vi "Complex Test.vi"() -> ()   [LabVIEW 2020, in "infolib.lvlib"]
doc: "Make a complex test of the library using premade tests/test.info."
uses:
  infolib.lvlib
  Get key polymorph parts/GetString.vi
  Add key polymorph parts/String.vi
  Get matrix polymorph parts/Get 2D String.vi
  Add matrix polymorph parts/2D String.vi
  Get key polymorph parts/GetTime Stamp.vi
  Add key polymorph parts/Time Stamp.vi
  Get matrix polymorph parts/Get 2D Time Stamp.vi
  Add matrix polymorph parts/2D Time Stamp.vi
  Get key polymorph parts/GetEXT.vi
  Add key polymorph parts/EXT.vi
  Get key polymorph parts/GetCXT.vi
  Add key polymorph parts/CXT.vi
  Get matrix polymorph parts/Get 2D EXT.vi
  Add matrix polymorph parts/2D EXT.vi
  Get matrix polymorph parts/Get 2D CXT.vi
  Add matrix polymorph parts/2D CXT.vi
  <vilib>/Utility/error.llb/Error Cluster From Error Code.vi
  <vilib>/ErrorRing/Error Ring.xnode
panel:
  in  "error limit for time":dbl=1e-06 format="%#_13g"
  in  "error limit for double":ext=1e-12
  in  "Test definitions and correct values":T1(array[cluster])=[{"k"="Test key, no value", "v"=[[""]], "t"="string", "s"=[]}, {"k"="Test key", "v"=[["A"]], "t"="string", "s"=[]}, {"k"="Test key, similar", "v"=[["B"]], "t"="string", "s"=[]}, {"k"="Test key, no spaces", "v"=[["C"]], "t"="string", "s"=[]}, {"k"="Test key, both spaces", "v"=[["D"]], "t"="string", "s"=[]}, {"k"="Test key, space left", "v"=[["E"]], "t"="string", "s"=[]}, {"k"="Test key, space right", "v"=[["F"]], "t"="string", "s"=[]}, {"k"="Test integer, 16 digits", "v"=[["1234567890123456"]], "t"="number", "s"=[]}, {"k"="Test floating point, 16 digits after decimal dot", "v"=[["0.1234567890123456"]], "t"="number", "s"=[]}, {"k"="Test floating point, 15 digits before decimal dot", "v"=[["123456789012345.6"]], "t"="number", "s"=[]}, {"k"="Test complex number", "v"=[["2.34+5.67i"]], "t"="compl. number", "s"=[]}, {"k"="Test imaginary number", "v"=[["8.90i"]], "t"="compl. number", "s"=[]}, {"k"="Test string, simple", "v"=[["test string"]], "t"="string", "s"=[]}, {"k"="Test string, nonletter characters", "v"=[["!@#$%^&*()-=[]{};'\"\\'\\\"\\:|,./<>?"]], "t"="string", "s"=[]}, {"k"="Test string, nonletter characters in key !@#$%^&*()-=[]{};'\"\\'\\\"\\:|,./<>?", "v"=[["in key"]], "t"="string", "s"=[]}, {"k"="Test string, UTF8 characters", "v"=[["\\u0159\\u0153\\u0414\\u03bc\\u03a9\\u211c\\u2111"]], "t"="string", "s"=[]}, {"k"="Test string, UTF8 characters in key \\u0159\\u0153\\u0414\\u03bc\\u03a9\\u211c\\u2111", "v"=[["in key"]], "t"="string", "s"=[]}, {"k"="Test time, no time zone", "v"=[["1014376332.123456"]], "t"="time", "s"=[]}, {"k"="Test time, with time zone, UTC", "v"=[["1014379932.123456"]], "t"="time", "s"=[]}, {"k"="Test time, with time zone, +10 minutes", "v"=[["1014379932.123456"]], "t"="time", "s"=[]}, {"k"="Test time, with time zone, +1 hour", "v"=[["1014379932.123456"]], "t"="time", "s"=[]}, {"k"="Test time, with time zone, -1 hour", "v"=[["1014379932.123456"]], "t"="time", "s"=[]}, {"k"="Test time, with time zone, +1:10", "v"=[["1014379932.123456"]], "t"="time", "s"=[]}, {"k"="Test time, with time zone, -1:10", "v"=[["1014379932.123456"]], "t"="time", "s"=[]}, {"k"="Test matrix, empty", "v"=[[""]], "t"="matrix number", "s"=[]}, {"k"="Test matrix, single value", "v"=[["1"]], "t"="matrix number", "s"=[]}, {"k"="Test matrix, single value, nonletter characters in key !@#$%^&*()-=[]{};'\"\\'\\\"\\:|,./<>?", "v"=[["2"]], "t"="matrix number", "s"=[]}, {"k"="Test matrix, single value, UTF8 characters in key  \\u0159\\u0153\\u0414\\u03bc\\u03a9\\u211c\\u2111", "v"=[["3"]], "t"="matrix number", "s"=[]}, {"k"="Test matrix, row numbers", "v"=[["4", "5", "6"]], "t"="matrix number", "s"=[]}, {"k"="Test matrix, column numbers", "v"=[["7"], ["8"], ["9"]], "t"="matrix number", "s"=[]}, {"k"="Test matrix", "v"=[["1.1", "2.1", "3.1"], ["4e4", "-5e5", "6e-6"], ["7.7e7", "8.123456789e1", "NaN"]], "t"="matrix number", "s"=[]}, {"k"="Test matrix complex", "v"=[["1.234", "2.345i", "3.456+4.567i"]], "t"="matrix compl. number", "s"=[]}, {"k"="Test matrix, mixed numbers and text for reading as numbers", "v"=[["1", "NaN", "2", "NaN"], ["3", "NaN", "4", "NaN"]], "t"="matrix number", "s"=[]}, {"k"="Test matrix, mixed numbers and text for reading as strings", "v"=[["11", "One", "12", "Two"], ["13", "Three", "14", "Four"]], "t"="matrix string", "s"=[]}, {"k"="Test matrix, mixed numbers and text with special characters read as numbers", "v"=[["1", "NaN", "2", "NaN"], ["3", "NaN", "4", "NaN"]], "t"="matrix number", "s"=[]}, {"k"="Test matrix, mixed numbers and text with special characters read as strings", "v"=[["11", "One;One", "12", "Two\"Two"], ["13", "Three;Three", "14", "Four\n                Four"]], "t"="matrix string", "s"=[]}, {"k"="Test matrix, time values", "v"=[["1014379932.123456", "1014383532.123456"], ["1014387132.123456", "1014390732.123456"]], "t"="matrix time", "s"=[]}, {"k"="Test matrix, lousy format and spaces", "v"=[["77", "8.8", "NaN"], ["NaN", "999", "10"], ["11", "12", "13"]], "t"="matrix number", "s"=[]}, {"k"="Key for section test", "v"=[["1"]], "t"="number", "s"=[""]}, {"k"="Key for section test", "v"=[["2"]], "t"="number", "s"=["Test section"]}, {"k"="Key for section test", "v"=[["3"]], "t"="number", "s"=["Test section", "Test subsection"]}, {"k"="Key for section test", "v"=[["4"]], "t"="number", "s"=["Test section", "Test subsection", "Test subsubsection"]}, {"k"="Key for section test", "v"=[["5"]], "t"="number", "s"=["Test section", "Test subsection", "Test subsubsection", "Test subsubsubsection"]}, {"k"="Key for section test", "v"=[["6"]], "t"="number", "s"=["Test section 2"]}, {"k"="Key for section test", "v"=[["7"]], "t"="number", "s"=["Test section 2", "Test section 2"]}, {"k"="Key for section test", "v"=[["8"]], "t"="number", "s"=["Test section 2", "Test section 2", "Test section 2"]}, {"k"="Key for section test", "v"=[["9"]], "t"="number", "s"=["Test section 2", "Test section 2", "Test section 2", "Test section 2"]}, {"k"="Key for section test", "v"=[["10"]], "t"="number", "s"=["Test section, nonletter characters in key !@#$%^&*()-=[]{};'\"\\'\\\"\\:|,./<>?"]}, {"k"="Key for section test", "v"=[["11"]], "t"="number", "s"=["Test section, UTF8 characters in key \\u0159\\u0153\\u0414\\u03bc\\u03a9\\u211c\\u2111"]}, {"k"="Key for section test", "v"=[["!@#$%^&*()-=[]{};'\"\\'\\\"\\:|,./<>?"]], "t"="section", "s"=["Test section, special characters inside"]}]
  in  "Do also tmp.info?":bool=TRUE
  in  "start:":i32
  in  "end:":i32=100
  out "tmp.info: all correct?":bool
  out "tmp.info: all keys found?":bool
  out "Results of testing":T2(array[cluster])
  out "test.info: all keys found?":bool
  out "test.info: all correct?":bool
  # "k: key, v: value of correct value, t: test type, s: section(s)"
  # "For details see \"tests/info_test.m\" and \"tests/test.info\"."
  # "Do not change values in the array without changing test.info and other testing scripts (infolib_test.m)!"
  # "First run from test.info"
  # "test index, test key, key found?, test correct?"
  # "Second run from generated tmp.info"
  # "For debugging: do tests only from index"
  # "to index"
  # "(inclusive), do tmp.info"
  # "<- To make full test, set values to 0 and 100 and check tmp.info."
  # "List of bad tests, with very small impact:\n15, 16, 27, 47, 48: LV cannot handle UTF8 characters\n43: fails if tests 47 and 48 are present in tmp.info, otherwise is ok.\n30: rounding error on 17th significant place\n34,:LV cannot handle proper csv: cell \"X;X\" is considered as two cells because LV do not know apostroph enclosing\n36: rounding error on 7th decimal place of time stamp"
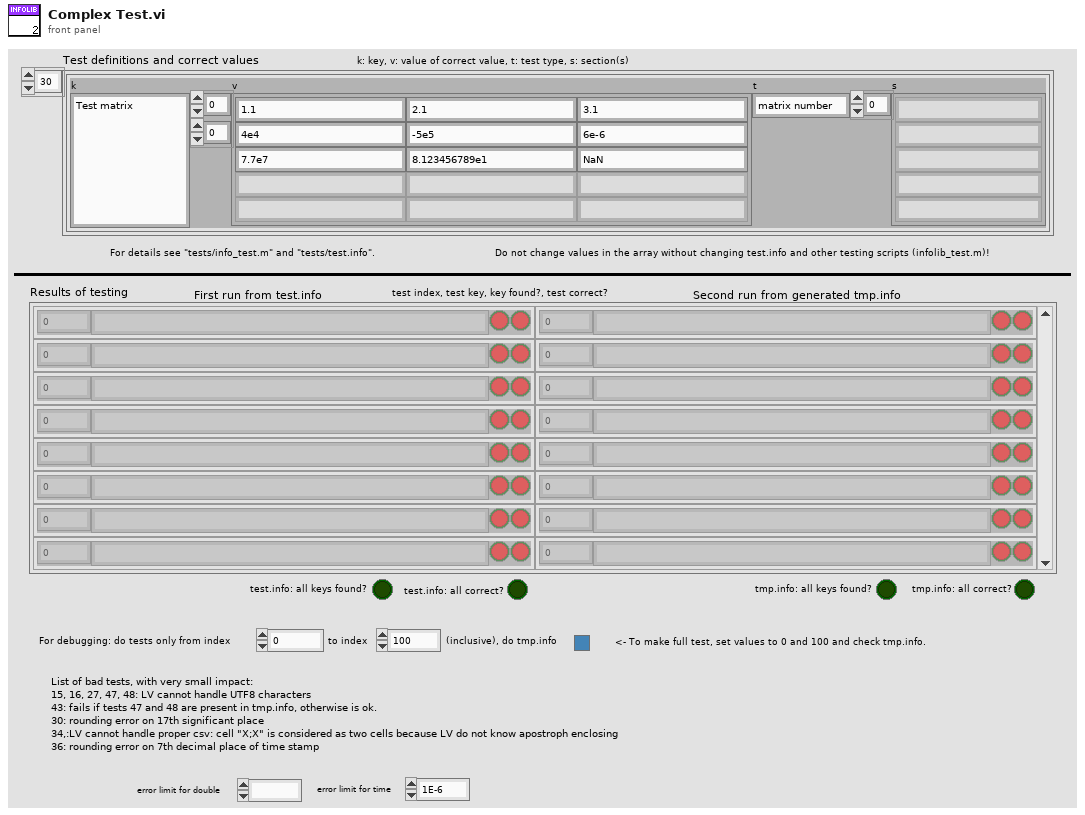
[diagram p1: front panel]
types:
  T1 = cluster{"k":string, "v":string[][], "t":string, "s":string[]}[]
  T2 = cluster{"index":i32, "key":string, "key found?":bool, "correct?":bool}[][]
  T3 = cluster{"index":i32, "key":string, "key found?":bool, "correct?":bool}
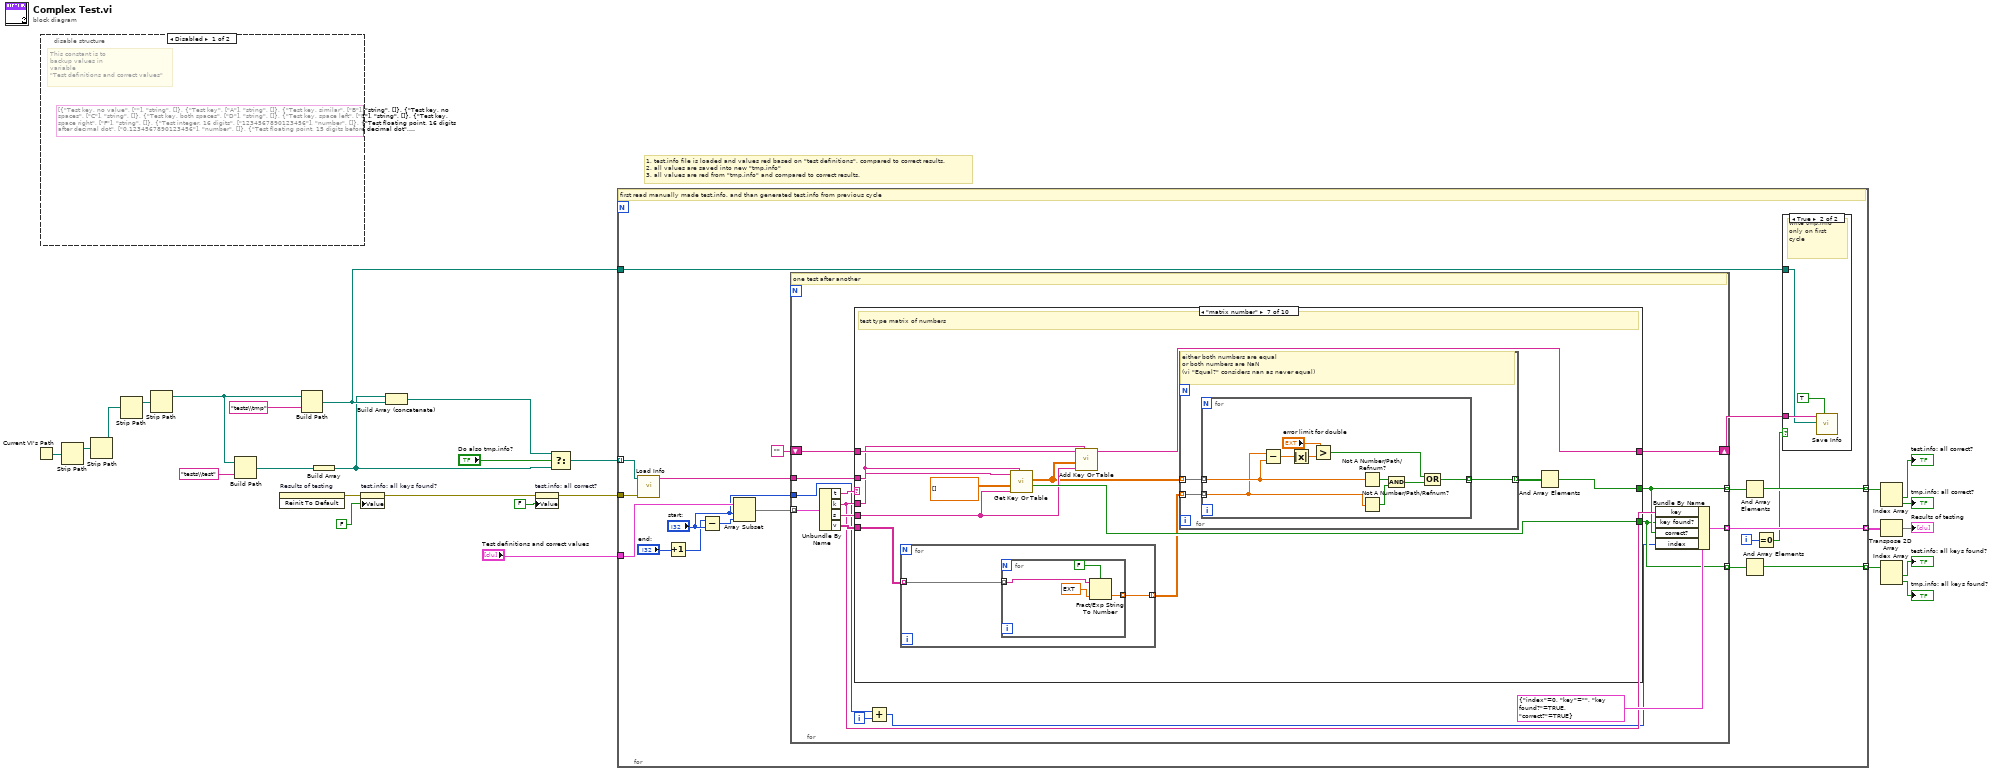
[diagram p0: block diagram]
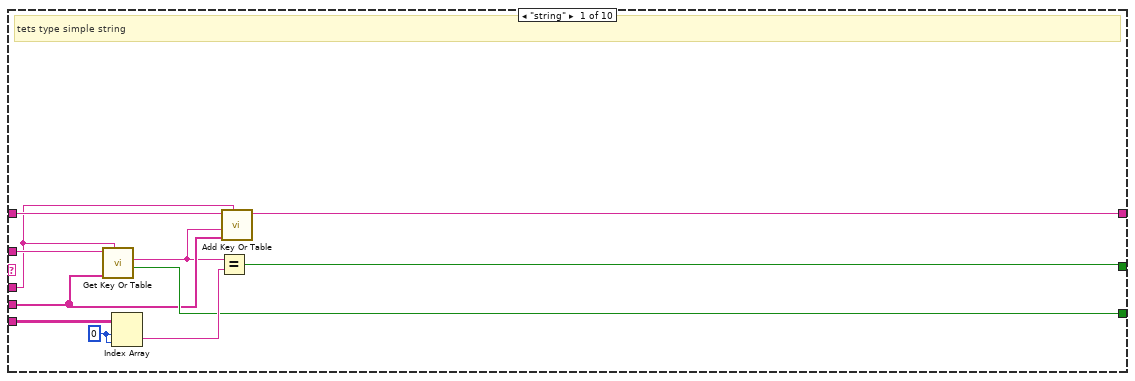
[diagram p3: hidden frame]
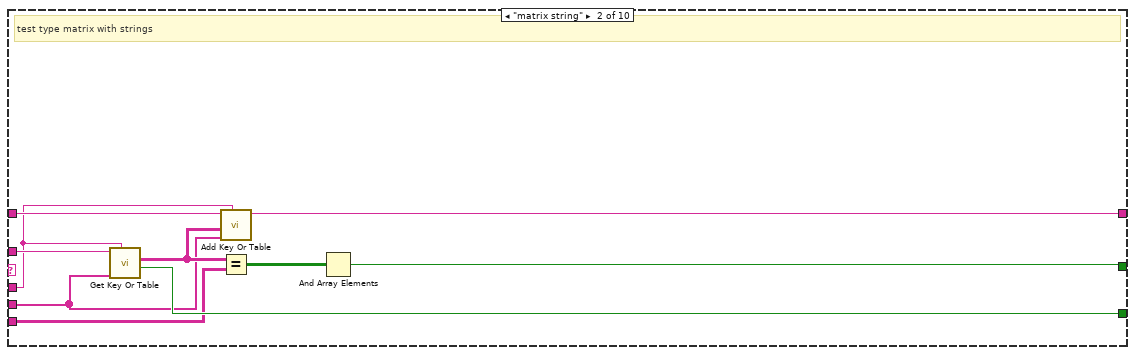
[diagram p4: hidden frame]
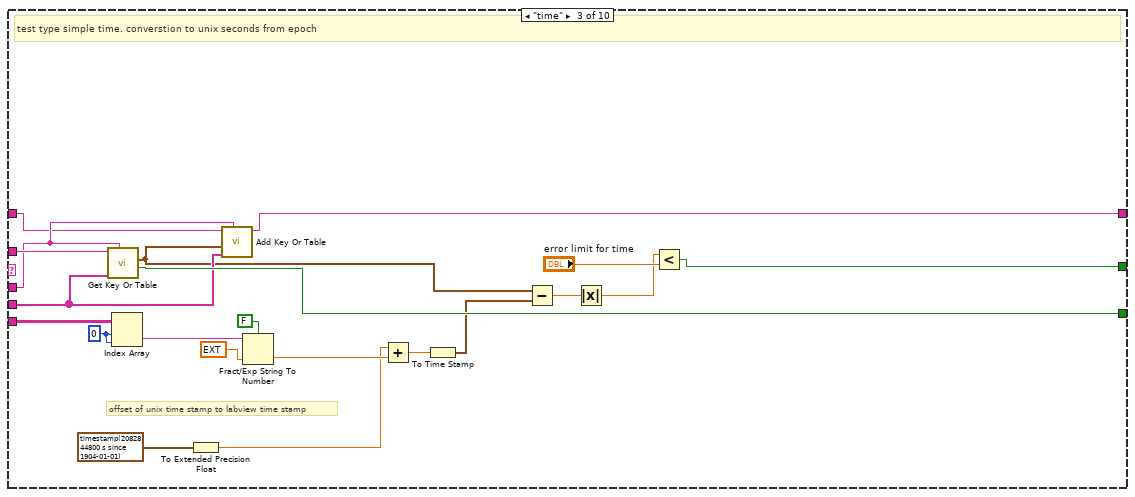
[diagram p5: hidden frame]
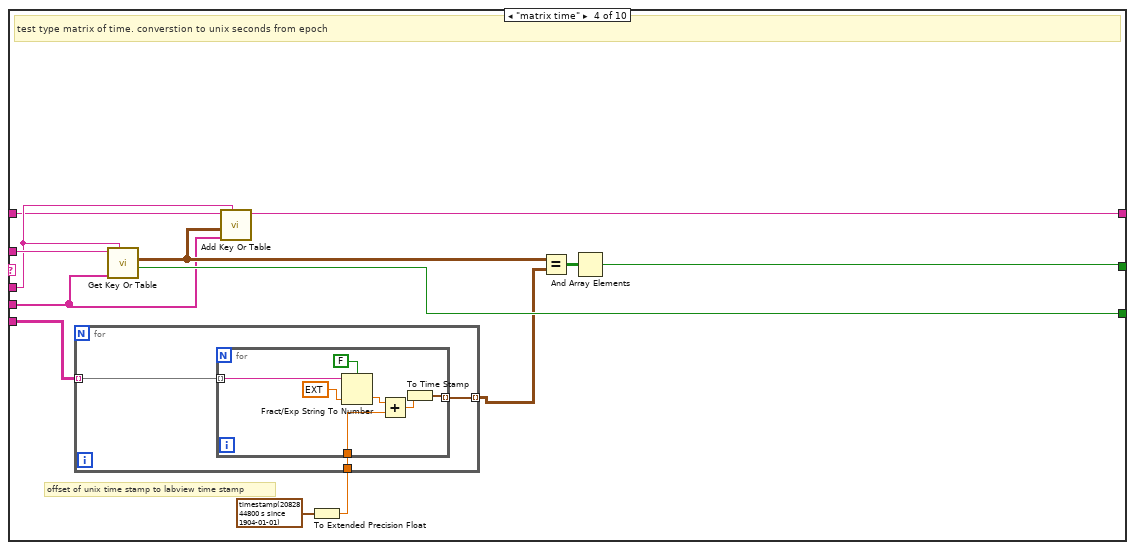
[diagram p6: hidden frame]
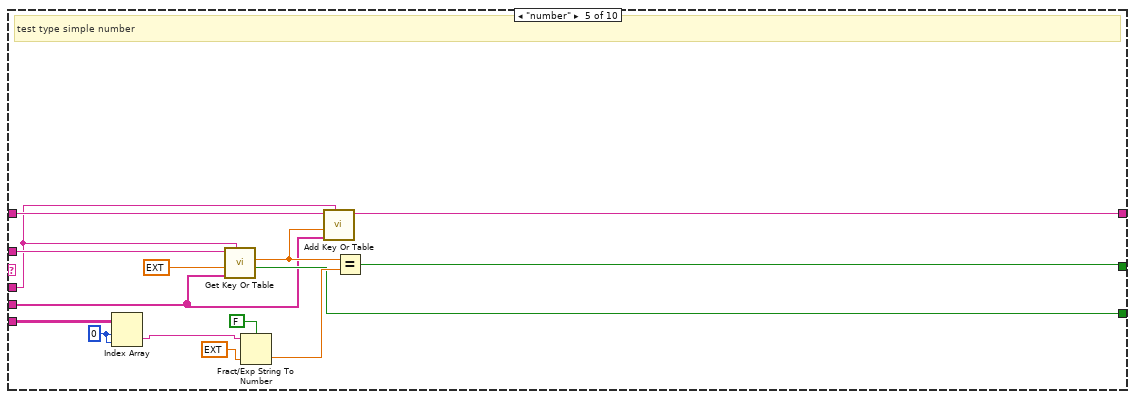
[diagram p7: hidden frame]
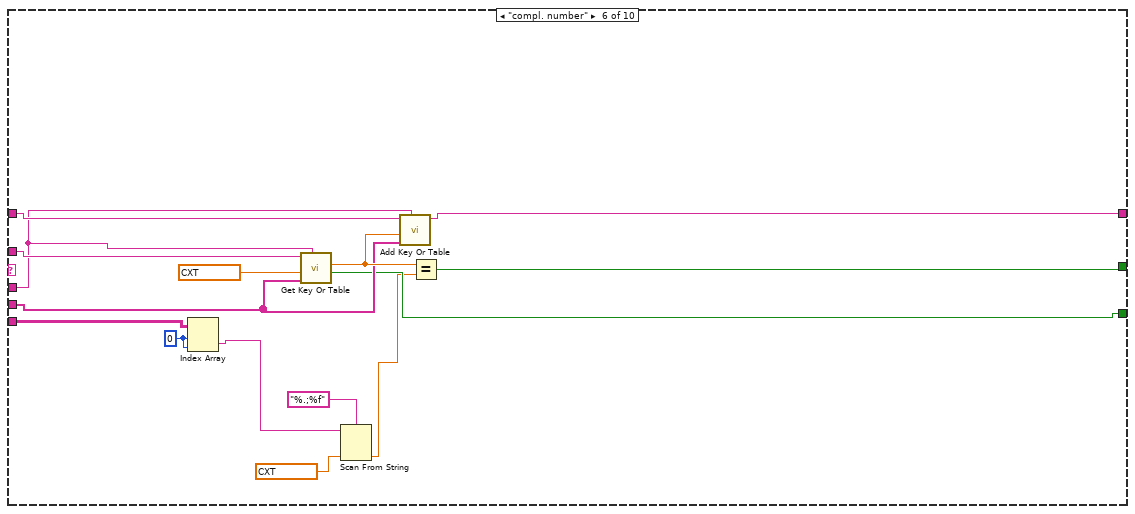
[diagram p8: hidden frame]
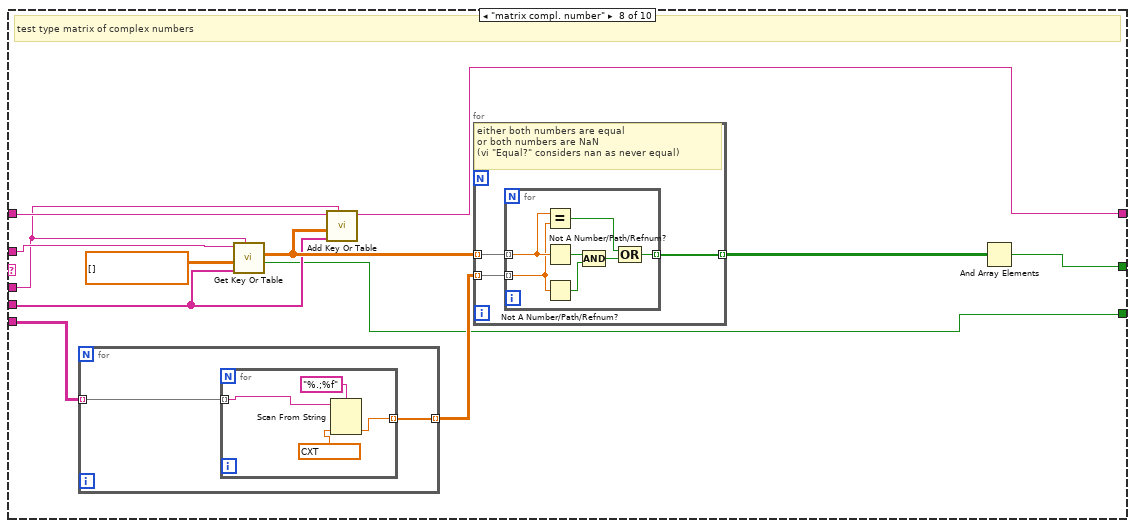
[diagram p9: hidden frame]
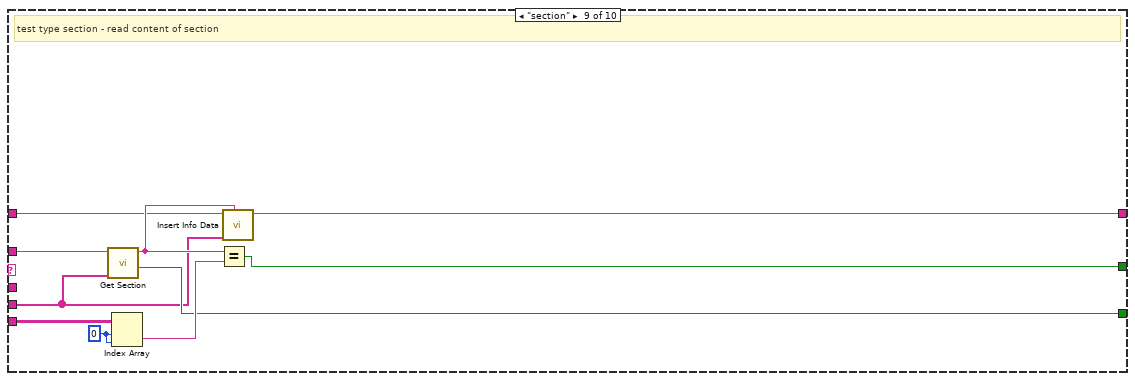
[diagram p10: hidden frame]
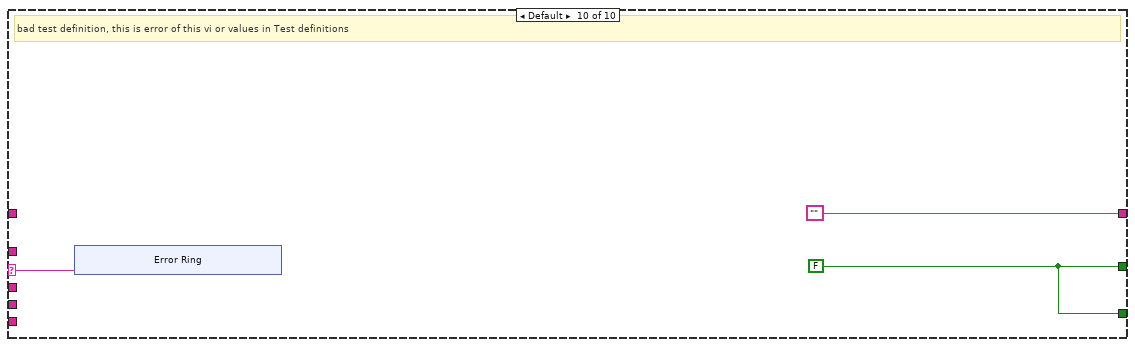
[diagram p11: hidden frame]
diagram:
  # "1, test.info file is loaded and values red based on \"test definitions\", compared to correct results.\n2, all values are saved into new \"tmp.info\"\n3, all values are red from \"tmp.info\" and compared to correct results."
  n1 = Current VI's Path() -> (path=w15:path)
  n2 = disable-structure shown="Disabled" {
    frame Disabled {
      (unwired) T1 [{"k"="Test key, no value", "v"=[[""]], "t"="string", "s"=[]}, {"k"="Test key", "v"=[["A"]], "t"="string", "s"=[]}, {"k"="Test key, similar", "v"=[["B"]], "t"="string", "s"=[]}, {"k"="Test key, no spaces", "v"=[["C"]], "t"="string", "s"=[]}, {"k"="Test key, both spaces", "v"=[["D"]], "t"="string", "s"=[]}, {"k"="Test key, space left", "v"=[["E"]], "t"="string", "s"=[]}, {"k"="Test key, space right", "v"=[["F"]], "t"="string", "s"=[]}, {"k"="Test integer, 16 digits", "v"=[["1234567890123456"]], "t"="number", "s"=[]}, {"k"="Test floating point, 16 digits after decimal dot", "v"=[["0.1234567890123456"]], "t"="number", "s"=[]}, {"k"="Test floating point, 15 digits before decimal dot", "v"=[["123456789012345.6"]], "t"="number", "s"=[]}, {"k"="Test complex number", "v"=[["2.34+5.67i"]], "t"="compl. number", "s"=[]}, {"k"="Test imaginary number", "v"=[["8.90i"]], "t"="compl. number", "s"=[]}, {"k"="Test string, simple", "v"=[["test string"]], "t"="string", "s"=[]}, {"k"="Test string, nonletter characters", "v"=[["!@#$%^&*()-=[]{};'\"\\'\\\"\\:|,./<>?"]], "t"="string", "s"=[]}, {"k"="Test string, nonletter characters in key !@#$%^&*()-=[]{};'\"\\'\\\"\\:|,./<>?", "v"=[["in key"]], "t"="string", "s"=[]}, {"k"="Test string, UTF8 characters", "v"=[["\\u0159\\u0153\\u0414\\u03bc\\u03a9\\u211c\\u2111"]], "t"="string", "s"=[]}, {"k"="Test string, UTF8 characters in key \\u0159\\u0153\\u0414\\u03bc\\u03a9\\u211c\\u2111", "v"=[["in key"]], "t"="string", "s"=[]}, {"k"="Test time, no time zone", "v"=[["1014376332.123456"]], "t"="time", "s"=[]}, {"k"="Test time, with time zone, UTC", "v"=[["1014379932.123456"]], "t"="time", "s"=[]}, {"k"="Test time, with time zone, +10 minutes", "v"=[["1014379932.123456"]], "t"="time", "s"=[]}, {"k"="Test time, with time zone, +1 hour", "v"=[["1014379932.123456"]], "t"="time", "s"=[]}, {"k"="Test time, with time zone, -1 hour", "v"=[["1014379932.123456"]], "t"="time", "s"=[]}, {"k"="Test time, with time zone, +1:10", "v"=[["1014379932.123456"]], "t"="time", "s"=[]}, {"k"="Test time, with time zone, -1:10", "v"=[["1014379932.123456"]], "t"="time", "s"=[]}, {"k"="Test matrix, empty", "v"=[[""]], "t"="matrix number", "s"=[]}, {"k"="Test matrix, single value", "v"=[["1"]], "t"="matrix number", "s"=[]}, {"k"="Test matrix, single value, nonletter characters in key !@#$%^&*()-=[]{};'\"\\'\\\"\\:|,./<>?", "v"=[["2"]], "t"="matrix number", "s"=[]}, {"k"="Test matrix, single value, UTF8 characters in key  \\u0159\\u0153\\u0414\\u03bc\\u03a9\\u211c\\u2111", "v"=[["3"]], "t"="matrix number", "s"=[]}, {"k"="Test matrix, row numbers", "v"=[["4", "5", "6"]], "t"="matrix number", "s"=[]}, {"k"="Test matrix, column numbers", "v"=[["7"], ["8"], ["9"]], "t"="matrix number", "s"=[]}, {"k"="Test matrix", "v"=[["1.1", "2.1", "3.1"], ["4e4", "-5e5", "6e-6"], ["7.7e7", "8.123456789e1", "NaN"]], "t"="matrix number", "s"=[]}, {"k"="Test matrix complex", "v"=[["1.234", "2.345i", "3.456+4.567i"]], "t"="matrix compl. number", "s"=[]}, {"k"="Test matrix, mixed numbers and text for reading as numbers", "v"=[["1", "NaN", "2", "NaN"], ["3", "NaN", "4", "NaN"]], "t"="matrix number", "s"=[]}, {"k"="Test matrix, mixed numbers and text for reading as strings", "v"=[["11", "One", "12", "Two"], ["13", "Three", "14", "Four"]], "t"="matrix string", "s"=[]}, {"k"="Test matrix, mixed numbers and text with special characters read as numbers", "v"=[["1", "NaN", "2", "NaN"], ["3", "NaN", "4", "NaN"]], "t"="matrix number", "s"=[]}, {"k"="Test matrix, mixed numbers and text with special characters read as strings", "v"=[["11", "One;One", "12", "Two\"Two"], ["13", "Three;Three", "14", "Four\n                Four"]], "t"="matrix string", "s"=[]}, {"k"="Test matrix, time values", "v"=[["1014379932.123456", "1014379932.123456+1*3600"], ["1014379932.123456+2*3600", "1014379932.123456+3*3600"]], "t"="matrix time", "s"=[]}, {"k"="Key for section test", "v"=[["1"]], "t"="number", "s"=[""]}, {"k"="Key for section test", "v"=[["2"]], "t"="number", "s"=["Test section"]}, {"k"="Key for section test", "v"=[["3"]], "t"="number", "s"=["Test section", "Test subsection"]}, {"k"="Key for section test", "v"=[["4"]], "t"="number", "s"=["Test section", "Test subsection", "Test subsubsection"]}, {"k"="Key for section test", "v"=[["5"]], "t"="number", "s"=["Test section", "Test subsection", "Test subsubsection", "Test subsubsubsection"]}, {"k"="Key for section test", "v"=[["6"]], "t"="number", "s"=["Test section 2"]}, {"k"="Key for section test", "v"=[["7"]], "t"="number", "s"=["Test section 2", "Test section 2"]}, {"k"="Key for section test", "v"=[["8"]], "t"="number", "s"=["Test section 2", "Test section 2", "Test section 2"]}, {"k"="Key for section test", "v"=[["9"]], "t"="number", "s"=["Test section 2", "Test section 2", "Test section 2", "Test section 2"]}, {"k"="Key for section test", "v"=[["10"]], "t"="number", "s"=["Test section, nonletter characters in key !@#$%^&*()-=[]{};'\"\\'\\\"\\:|,./<>?"]}, {"k"="Key for section test", "v"=[["11"]], "t"="number", "s"=["Test section, UTF8 characters in key \\u0159\\u0153\\u0414\\u03bc\\u03a9\\u211c\\u2111"]}, {"k"="Key for section test", "v"=[["!@#$%^&*()-=[]{};'\"\\'\\\"\\:|,./<>?"]], "t"="section", "s"=["Test section, special characters inside"]}] ("Test definitions and correct values")
      # "This constant is to\nbackup values in\nvariable\n\"Test definitions and correct values\""
    }
    frame Enabled {
    }
  }
  n3 = Strip Path(path=w15) -> (stripped path=w14:path)  [unwired: 1 out]
  n4 = Strip Path(path=w14) -> (stripped path=w13:path)  [unwired: 1 out]
  n5 = Strip Path(path=w13) -> (stripped path=w12:path)  [unwired: 1 out]
  n6 = Strip Path(path=w12) -> (stripped path=w11:path)  [unwired: 1 out]
  n7 = Build Path(base path=w11, name or relative path="tests\\test") -> (appended path=w3:path)
  n8 = invoke on="Results of testing" class="Arr (strict)" method="Reinit To Default"() -> (error out=w8:errorcluster)  [unwired: 3 in, 2 out]
  n9 = Build Path(base path=w11, name or relative path="tests\\tmp") -> (appended path=w7:path)
  n10 = Build Array(w3) -> (w2:path[])
  n11 = property on="test.info: all keys found?" class="Bool (strict)"(error in=w8, "Value"=FALSE ("All keys found?")) -> (error out=w27:errorcluster)  [unwired: 1 in, 1 out]
  n12 = Build Array (concatenate)(w2, w7) -> (w4:path[])
  n13 = property on="test.info: all correct?" class="Bool (strict)"(error in=w27, "Value"=FALSE ("All correct?")) -> (error out=w26:errorcluster)  [unwired: 1 in, 1 out]
  n14 = Select(t=w4, s="Do also tmp.info?", f=w2) -> (s? t:f=w6:path[])
  n15 = for {
    tunnel: "Test definitions and correct values" -> [w33]
    tunnel: w6 -> [w46] mode=indexing
    tunnel: w26 -> [w44]
    tunnel: [w43] -> w10 mode=indexing
    tunnel: [w41] -> w17 mode=indexing
    tunnel: [w39] -> w21 mode=indexing
    tunnel: w7 -> [w34]
    i -> [w37]
    # "first read manually made test.info, and than generated test.info from previous cycle"
    n16 = call "Load Info.vi"("error in"=w44, "filename"=w46) -> ("info data"=w45:string)  [unwired: 8 in, 1 out]
    n17 = Increment(x="end:") -> (x+1=w28:i32)
    n18 = Subtract(x=w28, y="start:") -> (x-y=w30:i32)
    n19 = Array Subset(array=w33, index="start:", length=w30) -> (w32:T1)
    n20 = for {
      tunnel: w32 -> [w64] mode=indexing
      tunnel: w45 -> [w63]
      tunnel: [w57] -> w43 mode=indexing
      tunnel: [w56] -> w42 mode=indexing
      tunnel: [w55] -> w40 mode=indexing
      shift-right: [w53] -> w35
      shift-left: "" -> [w54]
      tunnel: "start:" -> [w51]
      i -> [w52]
      # "one test after another"
      n21 = Unbundle By Name(w64) -> ("t"=w62:string, "k"=w58:string, "s"=w61:string[], "v"=w60:string[][])
      n22 = case shown="\"matrix number\"" w62 {
        selector: w62 -> [_ _ _ _ _ _ _ _ _ w230]
        tunnel: w58 -> [w67 w79 w97 w112 w135 w155 w164 w196 _ _]
        tunnel: w63 -> [w75 w85 w106 w119 w144 w156 w171 w197 w228 _]
        tunnel: w61 -> [w69 w77 w96 w109 w133 w153 w163 w195 w220 _]
        tunnel: w60 -> [w74 w83 w105 w116 w143 w154 w168 w194 w227 _]
        tunnel: [w72 w81 w88 w114 w142 w152 w167 w191 w224 w231] -> w56
        tunnel: [w71 w84 w104 w118 w138 w150 w170 w193 w223 w231] -> w55
        tunnel: w54 -> [w70 w80 w95 w111 w136 w157 w166 w198 w221 _]
        tunnel: [w66 w76 w94 w110 w132 w151 w165 w192 w219 ""] -> w53
        frame "string" {
          w65 = 0 ("index (row)")
          # "tets type simple string"
          n23 = call-poly "Get Key Or Table.vi"("key description"=w67, "sections"=w69, "info data"=w75) -> ("key found?"=w71:bool, "value"=w68:string)  [unwired: 5 in, 2 out]
          n24 = Index Array(array=w74, index (row)=w65, index (col)=w65) -> (element=w73:string)
          n25 = Equal?(x=w68, y=w73) -> (x = y?=w72:bool)
          n26 = call-poly "Add Key Or Table.vi"("key description"=w67, "sections"=w69, "string"=w68, "info data"=w70) -> ("info data out"=w66:string)  [unwired: 6 in, 1 out]
        }
        frame "matrix string" {
          # "test type matrix with strings"
          n27 = call-poly "Get Key Or Table.vi"("key description"=w79, "sections"=w77, "info data"=w85) -> ("key found?"=w84:bool, "value"=w78:string[][])  [unwired: 5 in, 2 out]
          n28 = call-poly "Add Key Or Table.vi"("key description"=w79, "sections"=w77, "string"=w78, "info data"=w80) -> ("info data out"=w76:string)  [unwired: 6 in, 1 out]
          n29 = Equal?(x=w78, y=w83) -> (x = y?=w82:bool[][])
          n30 = And Array Elements(Boolean array=w82) -> (logical AND=w81:bool)
        }
        frame "time" {
          w93 = 0 ("index (row)")
          # "offset of unix time stamp to labview time stamp"
          # "test type simple time. converstion to unix seconds from epoch"
          n31 = call-poly "Get Key Or Table.vi"("key description"=w97, "sections"=w96, "info data"=w106) -> ("key found?"=w104:bool, "value"=w90:timestamp)  [unwired: 5 in, 2 out]
          n32 = Index Array(array=w105, index (row)=w93, index (col)=w93) -> (element=w102:string)
          n33 = To Extended Precision Float(1:timestamp(2082844800 s since 1904-01-01)) -> (0:w100:ext)
          n34 = call-poly "Add Key Or Table.vi"("key description"=w97, "sections"=w96, "time stamp"=w90, "info data"=w95) -> ("info data out"=w94:string)  [unwired: 6 in, 1 out]
          n35 = Fract/Exp String To Number(use system decimal point (T)=FALSE, string=w102, default (0 dbl)=ext nan ("default (0 DBL)")) -> (number=w101:ext)  [unwired: 1 in, 1 out]
          n36 = Add(x=w100, y=w101) -> (x+y=w98:ext)
          n37 = To Time Stamp(1:w98) -> (0:w91:timestamp)
          n38 = Subtract(x=w90, y=w91) -> (x-y=w87:dbl)
          n39 = Absolute Value(x=w87) -> (abs(x)=w86:dbl)
          n40 = Less?(x=w86, y="error limit for time") -> (x < y?=w88:bool)
        }
        frame "matrix time" {
          # "offset of unix time stamp to labview time stamp"
          # "test type matrix of time. converstion to unix seconds from epoch"
          n41 = call-poly "Get Key Or Table.vi"("key description"=w112, "sections"=w109, "info data"=w119) -> ("key found?"=w118:bool, "value"=w113:timestamp[][])  [unwired: 5 in, 2 out]
          n42 = call-poly "Add Key Or Table.vi"("key description"=w112, "sections"=w109, "time stamp"=w113, "info data"=w111) -> ("info data out"=w110:string)  [unwired: 6 in, 1 out]
          n43 = To Extended Precision Float(1:timestamp(2082844800 s since 1904-01-01)) -> (0:w107:ext)
          n44 = for {
            tunnel: [w122] -> w108 mode=indexing
            tunnel: w116 -> [w121] mode=indexing
            tunnel: w107 -> [w120]
            n45 = for {
              tunnel: [w124] -> w122 mode=indexing
              tunnel: w121 -> [w128] mode=indexing
              tunnel: w120 -> [w123]
              n46 = Fract/Exp String To Number(use system decimal point (T)=FALSE, string=w128, default (0 dbl)=ext nan ("default (0 DBL)")) -> (number=w126:ext)  [unwired: 1 in, 1 out]
              n47 = Add(x=w126, y=w123) -> (x+y=w125:ext)
              n48 = To Time Stamp(1:w125) -> (0:w124:timestamp)
            }
          }
          n49 = Equal?(x=w113, y=w108) -> (x = y?=w115:bool[][])
          n50 = And Array Elements(Boolean array=w115) -> (logical AND=w114:bool)
        }
        frame "number" {
          w131 = 0 ("index (row)")
          # "test type simple number"
          n51 = Index Array(array=w143, index (row)=w131, index (col)=w131) -> (element=w141:string)
          n52 = call-poly "Get Key Or Table.vi"("key description"=w135, "sections"=w133, "numeric"=ext nan, "info data"=w144) -> ("key found?"=w138:bool, "value"=w134:ext)  [unwired: 4 in, 2 out]
          n53 = Fract/Exp String To Number(use system decimal point (T)=FALSE, string=w141, default (0 dbl)=ext nan ("default (0 DBL)")) -> (number=w140:ext)  [unwired: 1 in, 1 out]
          n54 = call-poly "Add Key Or Table.vi"("key description"=w135, "sections"=w133, "numeric"=w134, "info data"=w136) -> ("info data out"=w132:string)  [unwired: 6 in, 1 out]
          n55 = Equal?(x=w134, y=w140) -> (x = y?=w142:bool)
        }
        frame "compl. number" {
          w158 = 0 ("index (row)")
          n56 = Index Array(array=w154, index (row)=w158, index (col)=w158) -> (element=w147:string)
          n57 = call-poly "Get Key Or Table.vi"("key description"=w155, "sections"=w153, "numeric"=cxt nan+nani, "info data"=w156) -> ("key found?"=w150:bool, "value"=w159:cxt)  [unwired: 4 in, 2 out]
          n58 = Scan From String(format string="%.;%f", input string=w147, default 1=cxt nan+nani ("numeric")) -> (output 1=w146:cxt)  [unwired: 2 in, 3 out]
          n59 = call-poly "Add Key Or Table.vi"("key description"=w155, "sections"=w153, "numeric"=w159, "info data"=w157) -> ("info data out"=w151:string)  [unwired: 6 in, 1 out]
          n60 = Equal?(x=w159, y=w146) -> (x = y?=w152:bool)
        }
        frame "matrix number" {
          # "test type matrix of numbers"
          n61 = for {
            tunnel: w168 -> [w186] mode=indexing
            tunnel: [w185] -> w161 mode=indexing
            n62 = for {
              tunnel: w186 -> [w189] mode=indexing
              tunnel: [w188] -> w185 mode=indexing
              n63 = Fract/Exp String To Number(use system decimal point (T)=FALSE, string=w189, default (0 dbl)=ext nan ("default (0 DBL)")) -> (number=w188:ext)  [unwired: 1 in, 1 out]
            }
          }
          n64 = call-poly "Get Key Or Table.vi"("key description"=w164, "sections"=w163, "numeric"=ext[][] [], "info data"=w171) -> ("key found?"=w170:bool, "value"=w162:ext[][])  [unwired: 4 in, 2 out]
          n65 = call-poly "Add Key Or Table.vi"("key description"=w164, "sections"=w163, "numeric"=w162, "info data"=w166) -> ("info data out"=w165:string)  [unwired: 6 in, 1 out]
          n66 = for {
            tunnel: w162 -> [w174] mode=indexing
            tunnel: w161 -> [w173] mode=indexing
            tunnel: [w172] -> w160 mode=indexing
            # "either both numbers are equal\nor both numbers are NaN\n(vi \"Equal?\" considers nan as never equal)"
            n67 = for {
              tunnel: w174 -> [w180] mode=indexing
              tunnel: w173 -> [w179] mode=indexing
              tunnel: [w181] -> w172 mode=indexing
              n68 = Subtract(x=w179, y=w180) -> (x-y=w178:ext)
              n69 = Absolute Value(x=w178) -> (abs(x)=w177:ext)
              n70 = Greater?(x="error limit for double", y=w177) -> (0:w176:bool)
              n71 = Not A Number/Path/Refnum?(number/path/refnum=w180) -> (NaN/Path/Refnum?=w182:bool)
              n72 = Not A Number/Path/Refnum?(number/path/refnum=w179) -> (NaN/Path/Refnum?=w183:bool)
              n73 = Compound Arithmetic op=AND(w182, w183) -> (w184:bool)
              n74 = Compound Arithmetic op=OR(w176, w184) -> (w181:bool)
            }
          }
          n75 = And Array Elements(Boolean array=w160) -> (logical AND=w167:bool)
        }
        frame "matrix compl. number" {
          # "test type matrix of complex numbers"
          n76 = for {
            tunnel: w194 -> [w214] mode=indexing
            tunnel: [w213] -> w201 mode=indexing
            n77 = for {
              tunnel: w214 -> [w215] mode=indexing
              tunnel: [w216] -> w213 mode=indexing
              n78 = Scan From String(format string="%.;%f", input string=w215, default 1=cxt nan+nani ("numeric")) -> (output 1=w216:cxt)  [unwired: 2 in, 3 out]
            }
          }
          n79 = call-poly "Get Key Or Table.vi"("key description"=w196, "sections"=w195, "numeric"=cxt[][] [], "info data"=w197) -> ("key found?"=w193:bool, "value"=w202:cxt[][])  [unwired: 4 in, 2 out]
          n80 = call-poly "Add Key Or Table.vi"("key description"=w196, "sections"=w195, "numeric"=w202, "info data"=w198) -> ("info data out"=w192:string)  [unwired: 6 in, 1 out]
          n81 = for {
            tunnel: w202 -> [w205] mode=indexing
            tunnel: w201 -> [w204] mode=indexing
            tunnel: [w203] -> w200 mode=indexing
            # "either both numbers are equal\nor both numbers are NaN\n(vi \"Equal?\" considers nan as never equal)"
            n82 = for {
              tunnel: w205 -> [w212] mode=indexing
              tunnel: w204 -> [w211] mode=indexing
              tunnel: [w206] -> w203 mode=indexing
              n83 = Equal?(x=w212, y=w211) -> (x = y?=w207:bool)
              n84 = Not A Number/Path/Refnum?(number/path/refnum=w212) -> (NaN/Path/Refnum?=w208:bool)
              n85 = Not A Number/Path/Refnum?(number/path/refnum=w211) -> (NaN/Path/Refnum?=w209:bool)
              n86 = Compound Arithmetic op=AND(w208, w209) -> (w210:bool)
              n87 = Compound Arithmetic op=OR(w207, w210) -> (w206:bool)
            }
          }
          n88 = And Array Elements(Boolean array=w200) -> (logical AND=w191:bool)
        }
        frame "section" {
          w226 = 0 ("index (row)")
          # "test type section - read content of section"
          n89 = call "Get Section.vi"("sections"=w220, "info data"=w228) -> ("exist"=w223:bool, "section part"=w222:string)  [unwired: 7 in, 1 out]
          n90 = Index Array(array=w227, index (row)=w226, index (col)=w226) -> (element=w225:string)
          n91 = Equal?(x=w222, y=w225) -> (x = y?=w224:bool)
          n92 = call "Insert Info Data.vi"("info data to insert"=w222, "sections"=w220, "info data"=w221) -> ("info data out"=w219:string)  [unwired: 7 in, 1 out]
        }
        frame Default {
          w231 = FALSE
          # "bad test definition, this is error of this vi or values in Test definitions"
          n93 = xnode "Error Ring"("parameter 0"=w230) -> ()  [unwired: 1 out]
        }
      }
      n94 = Add(x=w51, y=w52) -> (x+y=w50:i32)
      n95 = Bundle By Name(cluster=T3 {"index"=0, "key"="", "key found?"=TRUE, "correct?"=TRUE}, "key"=w58, "key found?"=w55, "correct?"=w56, "index"=w50) -> (w57:T3)
    }
    n96 = And Array Elements(Boolean array=w42) -> (logical AND=w41:bool)
    n97 = And Array Elements(Boolean array=w40) -> (logical AND=w39:bool)
    n98 = Equal To 0?(x=w37) -> (x = 0?=w36:bool)
    n99 = case shown="True" w36 {
      tunnel: w35 -> [_ w49]
      tunnel: w34 -> [_ w47]
      frame False {
      }
      frame True {
        # "write tmp.info\nonly on first\ncycle"
        n100 = call "Save Info.vi"("Overwrite? (T)"=TRUE, "filename"=w47, "info data"=w49) -> ()  [unwired: 8 in, 1 out]
      }
    }
  }
  n101 = Index Array(array=w17) -> (element #1=→"test.info: all correct?":bool, element #2=→"tmp.info: all correct?":bool)  [unwired: 2 in]
  n102 = Transpose 2D Array(2D array=w10) -> (transposed array=→"Results of testing":T2)
  n103 = Index Array(array=w21) -> (element #1=→"test.info: all keys found?":bool, element #2=→"tmp.info: all keys found?":bool)  [unwired: 2 in]
